vi "Add Report Information.vi"(8 "error in (no error)":errorcluster, 10 "Report Information.lvclass":refnum<class "Report Information.lvclass">, 11 "Report in":refnum<class "Report.lvclass">) -> (0 "error out":errorcluster, 3 "Report out":refnum<class "Report.lvclass">)   [LabVIEW 2015, in "Report.lvclass"]
doc: "This VI takes an entire Result Information object and saves it to a local object for writing to disk later."
uses:
  Report.lvclass
  Report Information/Report Information.lvclass
  Report.lvclass/Report.ctl
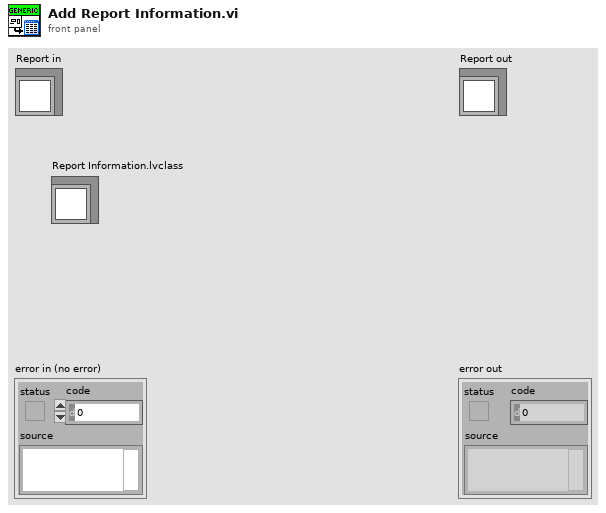
[diagram p1: front panel]
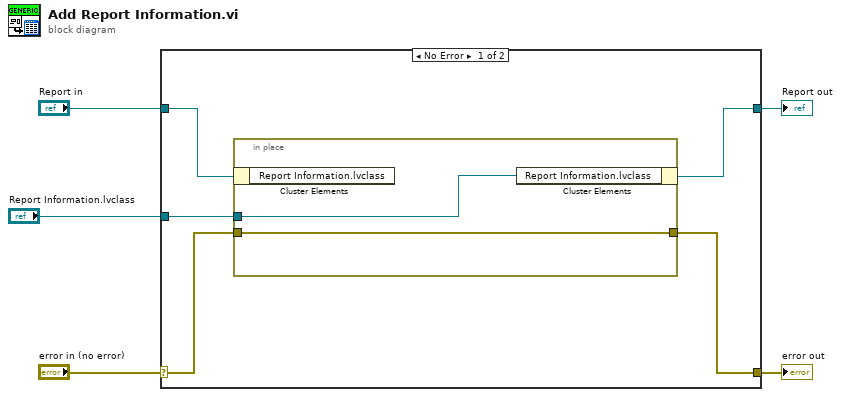
[diagram p0: block diagram]
diagram:
  n1 = case shown="No Error" "error in (no error)" {
    selector: "error in (no error)" -> [w9 w14]
    tunnel: [w8 w14] -> w4
    tunnel: [w7 w13] -> w2
    tunnel: "Report in" -> [w10 w13]
    tunnel: "Report Information.lvclass" -> [w6 _]
    frame No Error {
      n2 = in-place {
        in-place-border: w9 -> [w12]
        in-place-border: w6 -> [w11]
        in-place-border: [w12] -> w8
        n3 = in-place-cluster #1(w10) -> ()  [unwired: 1 out]
        n4 = in-place-cluster #1("Report Information.lvclass"=w11) -> (w7:refnum<class "Report.lvclass">)
      }
    }
    frame Error {
    }
  }
  "error out" <- w4
  "Report out" <- w2
